vi "Setup DCPower Voltage Sequence.vi"(7 "Channel Groups?":bool, 8 "error in (no error)":errorcluster, 9 "Parameters for Sequence":T1={"Supplies"=[], "Limit"=0.0, "Aperture Time"=0.0, "Settling Time"=0.0, "Sense"=1008, "Transient Response"=1041} {"Transient Response" items=["Slow"=1041, "Normal"=1038, "Fast"=1039, "Custom"=1042]; "Sense" items=["Local"=1008, "Remote"=1009]}, 10 "Channel List":string caption="channel name", 11 "DCPower Handle In":refnum<k15>) -> (0 "error out":errorcluster, 3 "DCPower Handle Out":refnum<k15>)   [LabVIEW 2021, in "PMIC Common.lvlib"]
uses:
  PMIC Common.lvlib
  <instrlib>/niDCPower/nidcpower.llb/niDCPower Source Mode.ctl
  <instrlib>/niDCPower/nidcpower.llb/niDCPower Output Function.ctl
  DCPower Parameters for Sequence.ctl
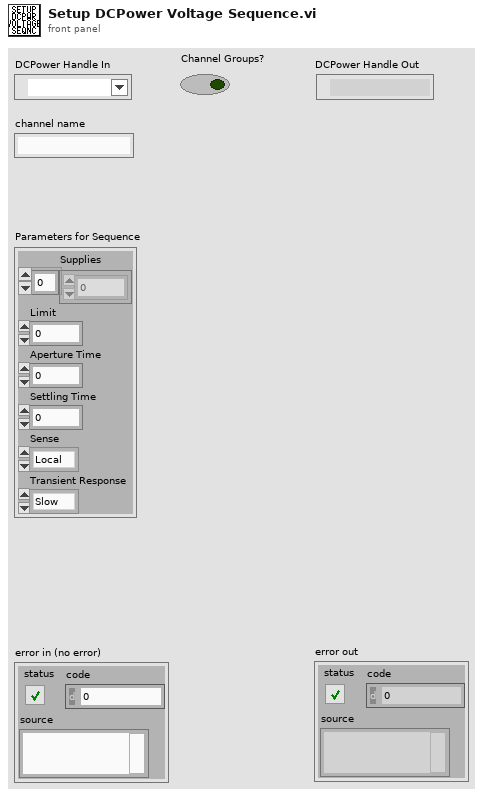
[diagram p1: front panel]
types:
  T1 = typedef "PMIC Common.lvlib/DCPower Parameters for Sequence.ctl" = cluster{"Supplies":dbl[], "Limit":dbl, "Aperture Time":dbl, "Settling Time":dbl, "Sense":i32, "Transient Response":i32}
  T2 = typedef "niDCPower Output Function.ctl" = i32
  T3 = typedef "niDCPower Source Mode.ctl" = i32
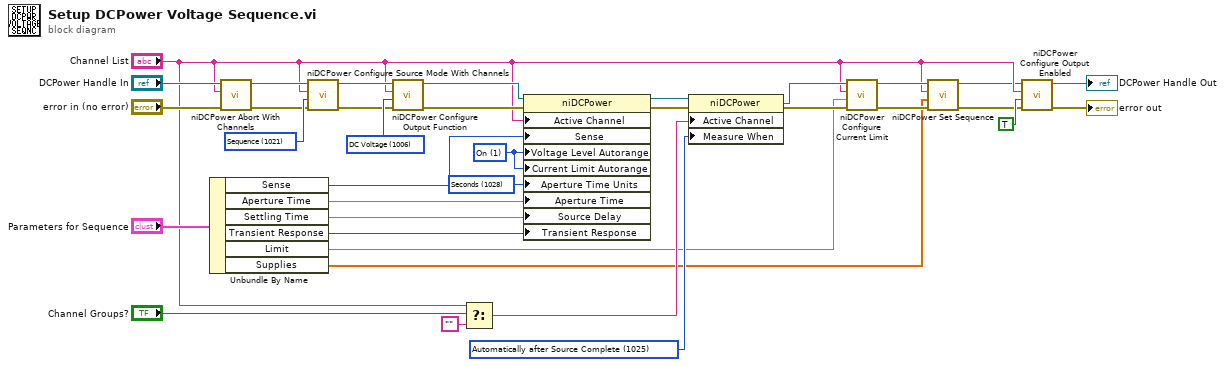
[diagram p0: block diagram]
diagram:
  w17 = 1028 items=["Seconds"=1028, "Power Line Cycles"=1029] ("Measurement:Aperture Time Units")
  w19 = 1025 items=["Automatically after Source Complete"=1025, "On Demand"=1026, "On Measure Trigger"=1027] ("Measurement:Advanced:Measure When")
  w27 = 1 items=["Off", "On"] ("DC Voltage:Voltage Level Autorange")
  w31 = T2 1006 items=["DC Voltage"=1006, "DC Current"=1007, "Pulse Voltage"=1049, "Pulse Current"=1050] ("output function")
  w30 = T3 1021 items=["Single Point"=1020, "Sequence"=1021] ("source mode")
  n1 = Unbundle By Name("Parameters for Sequence") -> ("Sense"=w15:i32, "Aperture Time"=w14:dbl, "Settling Time"=w13:dbl, "Transient Response"=w12:i32, "Limit"=w7:dbl, "Supplies"=w3:dbl[])
  n2 = call <instrlib>:"niDCPower Abort With Channels.vi"("error in (no error)"="error in (no error)", "channel name"="Channel List", "instrument handle"="DCPower Handle In") -> ("error out"=w24:errorcluster, "instrument handle out"=w25:refnum<k15>)  [unwired: 7 in]
  n3 = call <instrlib>:"niDCPower Configure Source Mode With Channels.vi"("error in (no error)"=w24, "source mode"=w30, "channel name"="Channel List", "instrument handle"=w25) -> ("error out"=w28:errorcluster, "instrument handle out"=w29:refnum<k15>)  [unwired: 6 in]
  n4 = call <instrlib>:"niDCPower Configure Output Function.vi"("error in (no error)"=w28, "output function"=w31, "channel name"="Channel List", "instrument handle"=w29) -> ("error out"=w35:errorcluster, "instrument handle out"=w34:refnum<k15>)  [unwired: 6 out]
  n5 = Select(t="Channel List", s="Channel Groups?", f="") -> (s? t:f=w20:string)
  n6 = property class="niDCPower"(reference=w34, error in=w35, "Active Channel"="Channel List", "Sense"=w15, "Voltage Level Autorange"=w27, "Current Limit Autorange"=w27, "Aperture Time Units"=w17, "Aperture Time"=w14, "Source Delay"=w13, "Transient Response"=w12) -> (reference out=w32:refnum<k15>, error out=w33:errorcluster)
  n7 = property class="niDCPower"(reference=w32, error in=w33, "Active Channel"=w20, "Measure When"=w19) -> (reference out=w9:refnum<k15>, error out=w8:errorcluster)
  n8 = call <instrlib>:"niDCPower Configure Current Limit.vi"("error in (no error)"=w8, "current limit"=w7, "channel name"="Channel List", "instrument handle"=w9) -> ("error out"=w5:errorcluster, "instrument handle out"=w6:refnum<k15>)  [unwired: 6 in]
  n9 = call <instrlib>:"niDCPower Set Sequence.vi"("error in (no error)"=w5, "values"=w3, "channel name"="Channel List", "instrument handle"=w6) -> ("error out"=w1:errorcluster, "instrument handle out"=w2:refnum<k15>)  [unwired: 6 in]
  n10 = call <instrlib>:"niDCPower Configure Output Enabled.vi"("error in (no error)"=w1, "output enabled"=TRUE, "channel name"="Channel List", "instrument handle"=w2) -> ("error out"=→"error out":errorcluster, "instrument handle out"=→"DCPower Handle Out":refnum<k15>)  [unwired: 6 in]
